vi "UI(Simple).vi"() -> (0 "error out":errorcluster)   [LabVIEW 2017, in "UI.lvlib"]
doc: "The Queued Message Handler of a Worker."
uses:
  UI.lvlib
  _support/UI State.ctl
  1af51285-6659-428e-9c15-de70f1a207c9.vi
  1756710f-d813-4077-a3f9-6f06171a4225.vi
  b1498353-a107-4479-98d0-7e76c0451ff6.vi
  242d01f8-d211-4c25-bb6c-8191a2acbe42.vi
  <userlib>/_NEVSTOP/Communicable State Machine(CSM)/_Polymophic/Add State(s) to Queue By BOOL(Element).vi
  <userlib>/_NEVSTOP/Communicable State Machine(CSM)/AdvanceAPI/CSM - Revert Arguments-Safe String.vi
  <userlib>/_NEVSTOP/Communicable State Machine(CSM)/AdvanceAPI/CSM - Make String Arguments Safe.vi
  <userlib>/_NEVSTOP/Communicable State Machine(CSM)/AdvanceAPI/CSM - Break Down Multiple States String.vi
  <userlib>/_NEVSTOP/Communicable State Machine(CSM)/AdvanceAPI/CSM - Keywords.vi
  <userlib>/_NEVSTOP/Communicable State Machine(CSM)/addons/INI-Static-Variable-Support/_Support/instances/_CSM - Read File Logger Configuration - v1.0.vi
  <userlib>/_NEVSTOP/Communicable State Machine(CSM)/_Shared/Trim Single-line Text.vi
  <userlib>/_NEVSTOP/Communicable State Machine(CSM)/addons/API-String-Arugments-Support/_Support/Convert API String Arguments to Data(variant).vi
  <userlib>/_NEVSTOP/Communicable State Machine(CSM)/addons/API-String-Arugments-Support/_Support/Query Data as API String Arguments(variant).vi
  <userlib>/_NEVSTOP/Communicable State Machine(CSM)/addons/MassData-Parameter/_support/FGV-MassData.vi
  Acquisition/Acquisition.lvlib
  Logging/Logging.lvlib
  <userlib>/_NEVSTOP/Communicable State Machine(CSM)/Communicable State Machine.lvlib
  <userlib>/_NEVSTOP/Communicable State Machine(CSM)/addons/MassData-Parameter/CSM MassData Parameter Support.lvlib
  <userlib>/_NEVSTOP/Communicable State Machine(CSM)/addons/INI-Static-Variable-Support/INI-Static-Variable-Support.lvlib
  <userlib>/_NEVSTOP/Communicable State Machine(CSM)/addons/Logger/CSM File Logger.lvlib
  <userlib>/_NEVSTOP/Communicable State Machine(CSM)/addons/Watchdog/CSM Watchdog.lvlib
  <userlib>/_NEVSTOP/Communicable State Machine(CSM)/_Polymophic/Build Synchronous Message with Arguments.vi
panel:
  out "WaveformGraph":waveform(dbl)[](graph)
  in  "Settings":bool
  in  "Start":bool
  in  "Stop":bool
  out "Status":string
  in  "Exit":bool
  # "Continuous Measurement and Data Logger - CSM Version"
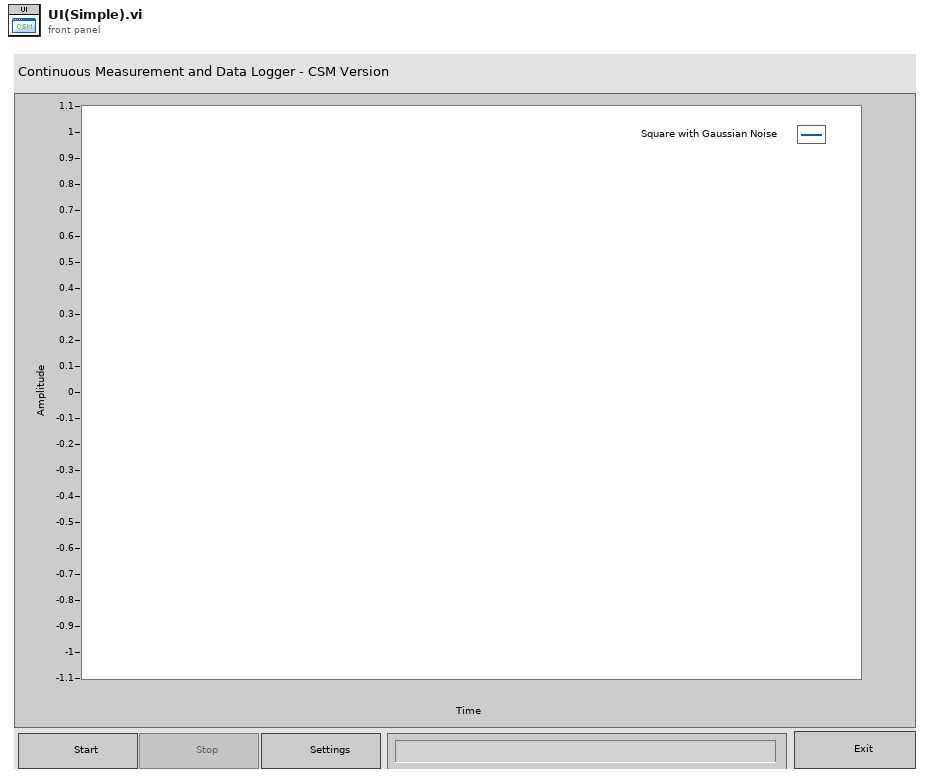
[diagram p1: front panel]
types:
  T1 = cluster{"Enable":bool, "Limit":cluster{"FileSize":i64, "FileNum":i32}, "Timestamp.Format":string, "AutoExit":bool}
  T2 = enum32{"Invalid", "Standard", "Closed", "Hidden", "Minimized", "Maximized"}
  T3 = enum32{"invalid app kind", "Development System", "Run Time System", "Student Edition", "Embedded LabVIEW", "Evaluation", "Custom"}
  T4 = typedef "UI.lvlib/UI State.ctl" = enum16{"Idle", "Acquiring and Logging", "Waiting for Exit", "Waiting for Exit (Acq Stopped)", "Waiting for Exit (Log Stopped)", "Waiting for Stop", "Waiting for Stop (Acq Stopped)", "Waiting for Stop (Log Stopped)"}
  T5 = enum32{"Invalid", "Default", "Floating", "Floating/Auto-Hide", "Modal"}
  T6 = typedef "Communicable State Machine.lvlib/_CSM_Response Source Message.ctl" = cluster{"‘State":string, "’Arguments":string, "’Error":errorcluster}
  T7 = cluster{"Current VI Reference":refnum<vi>, "Close Panel on Exit?":bool}
  T8 = cluster{"Core":cluster{"Current VI Reference":refnum<vi>, "Close Panel on Exit?":bool}, "UI Refs":cluster{"Start Ref":refnum<vi>, "Stop Ref":refnum<vi>, "Settings Ref":refnum<vi>, "Exit Ref":refnum<vi>, "Status Ref":refnum<vi>, "Data Ref":refnum<vi>, "Data Source Ref":refnum<vi>}, "State":T4, "Relationships":string}
  T9 = cluster{"Start Ref":refnum<vi>, "Stop Ref":refnum<vi>, "Settings Ref":refnum<vi>, "Exit Ref":refnum<vi>, "Status Ref":refnum<vi>, "Data Ref":refnum<vi>, "Data Source Ref":refnum<vi>}
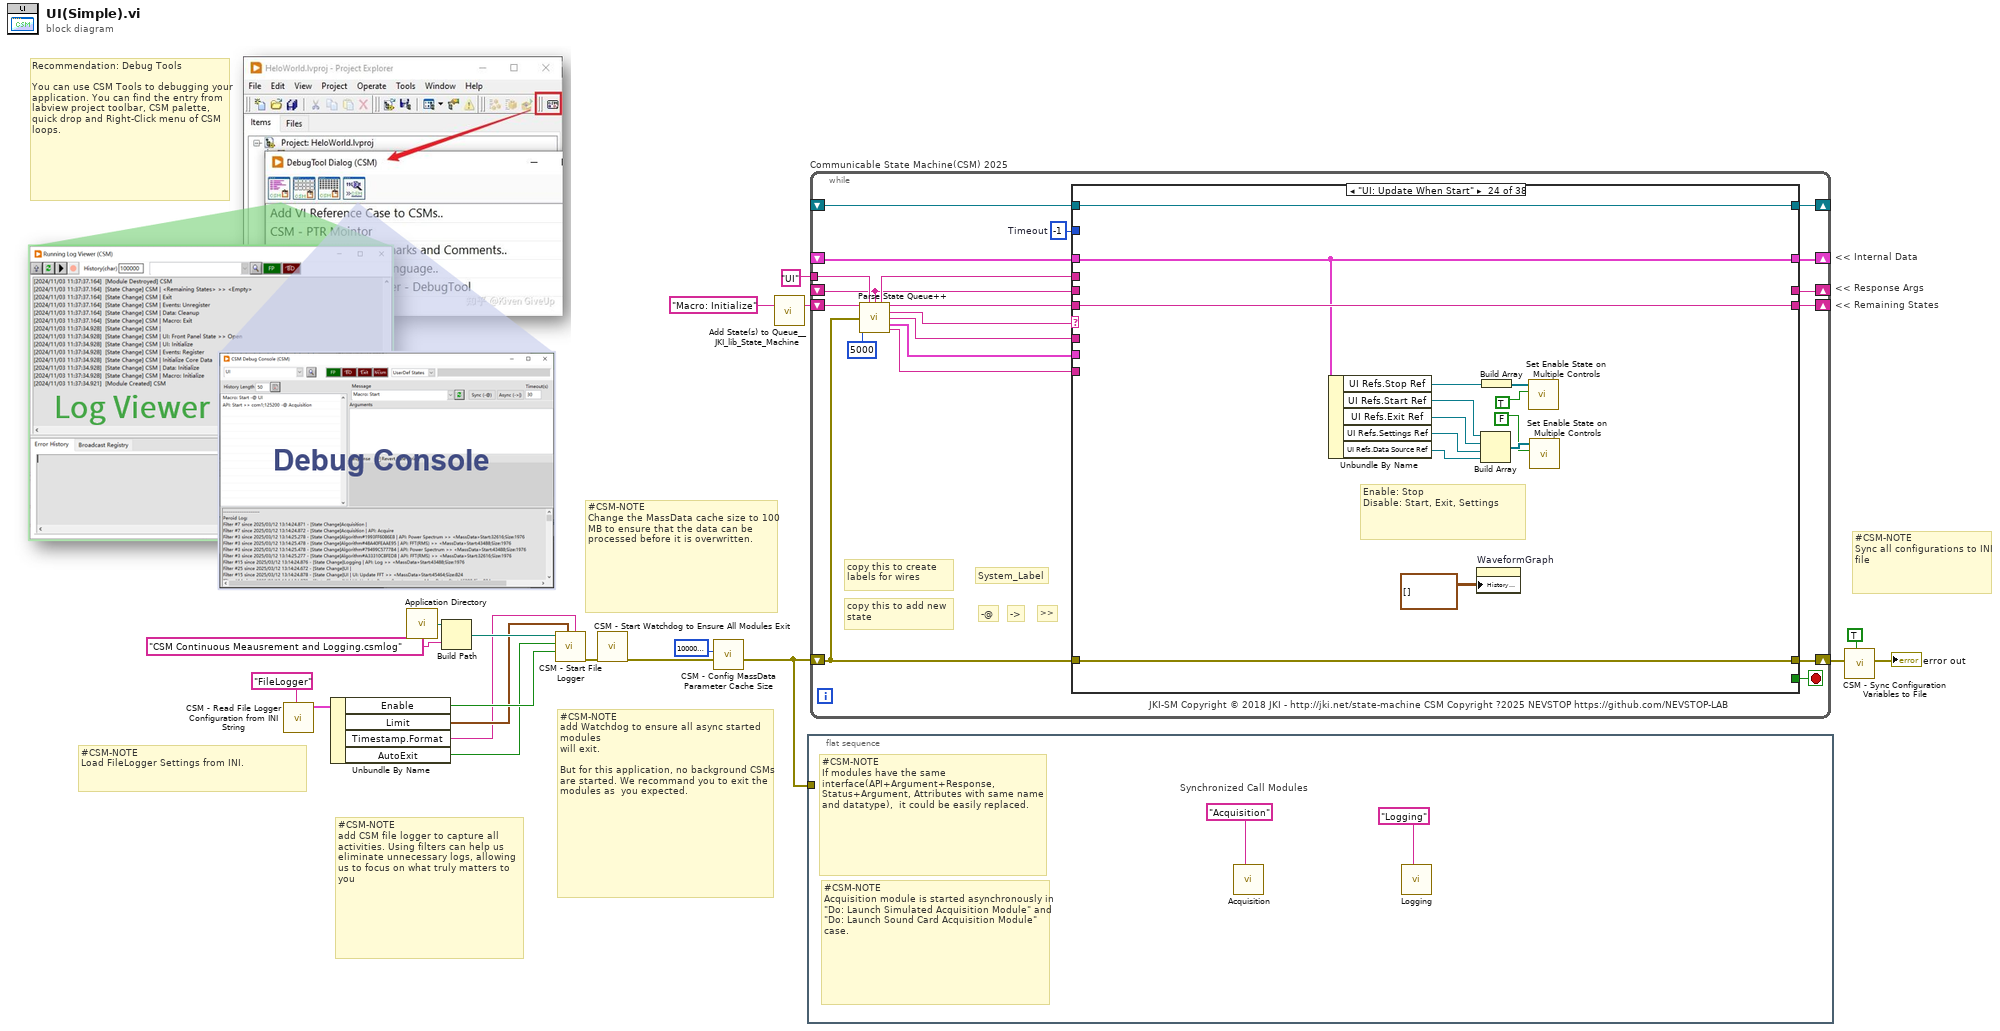
[diagram p0: block diagram]
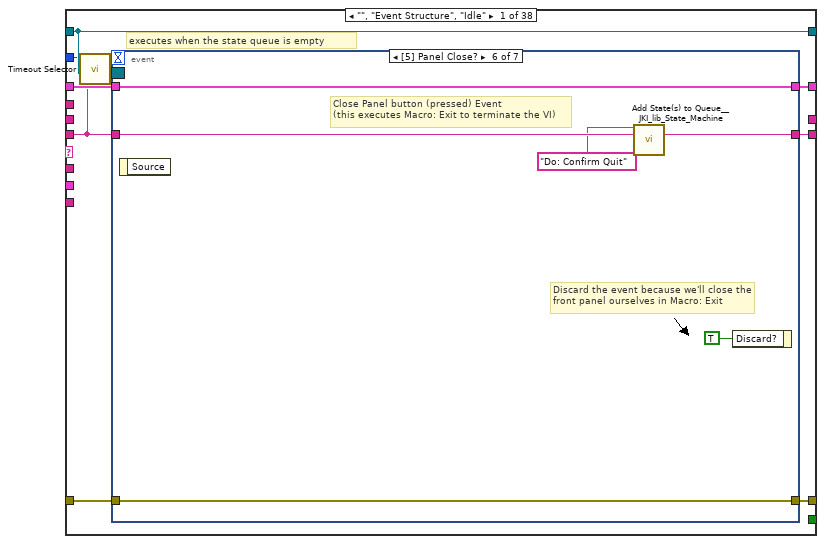
[diagram p2: hidden frame]
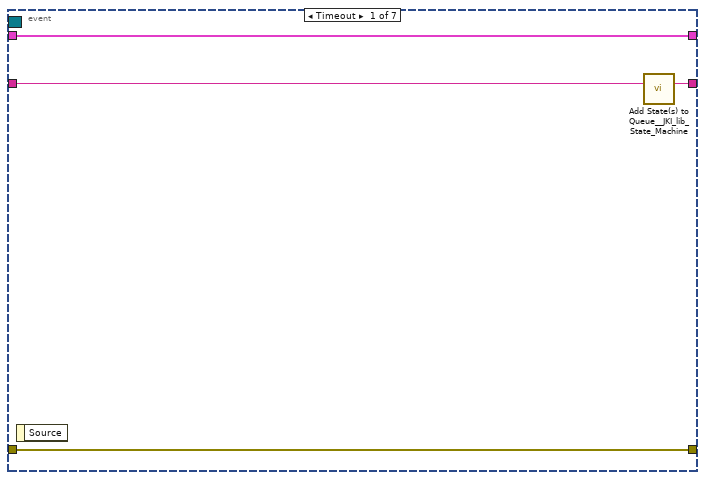
[diagram p3: hidden frame]
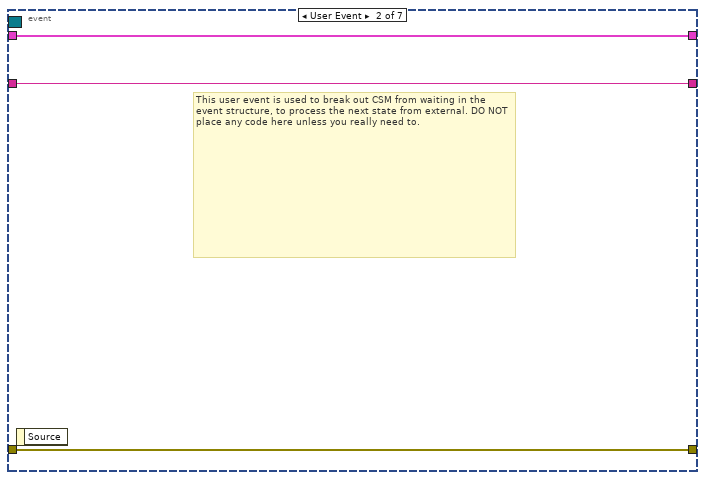
[diagram p4: hidden frame]
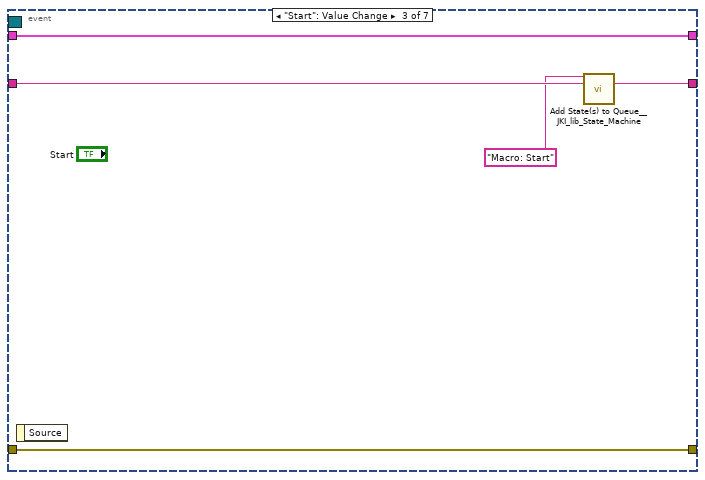
[diagram p5: hidden frame]
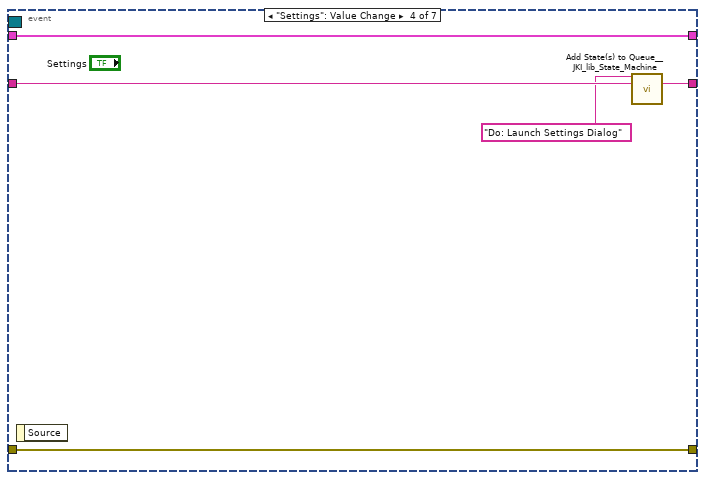
[diagram p6: hidden frame]
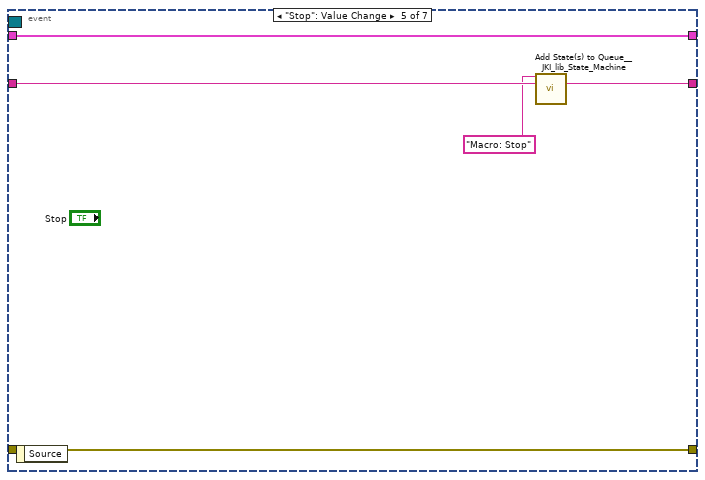
[diagram p7: hidden frame]
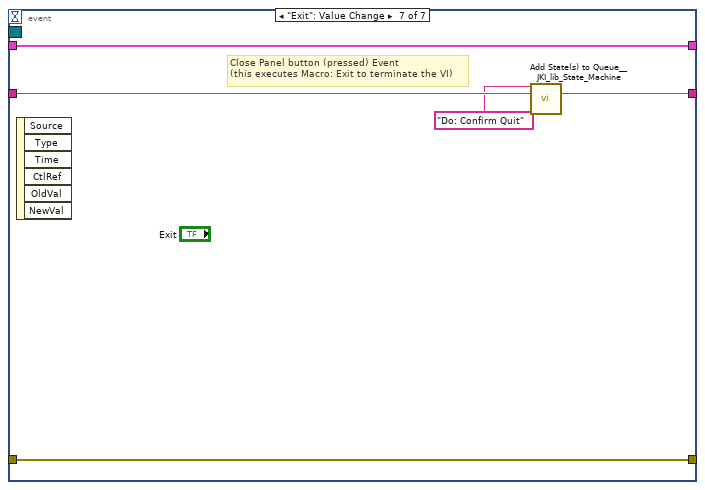
[diagram p8: hidden frame]
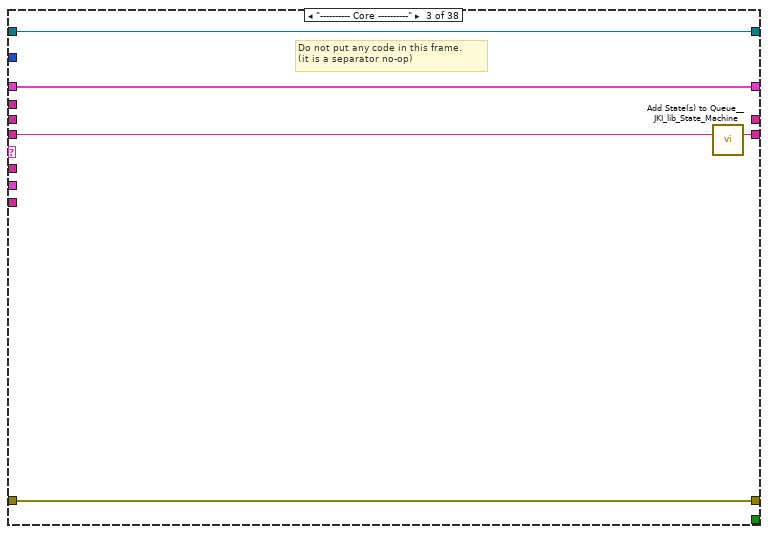
[diagram p10: hidden frame]
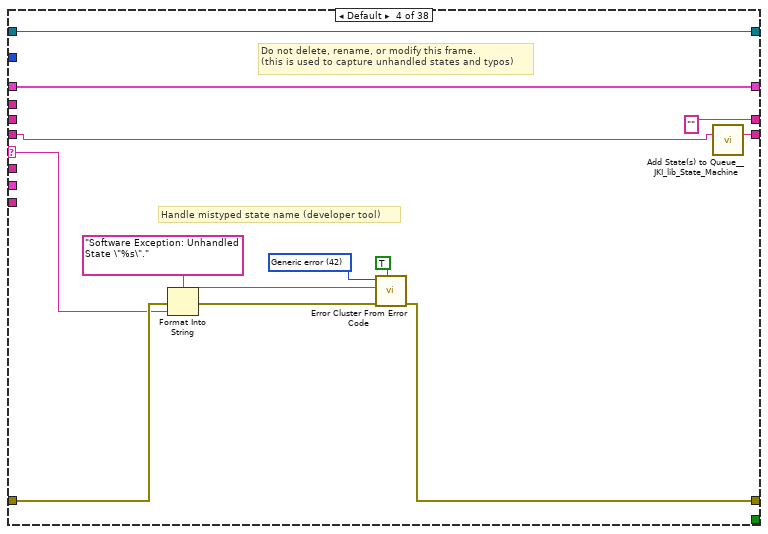
[diagram p11: hidden frame]
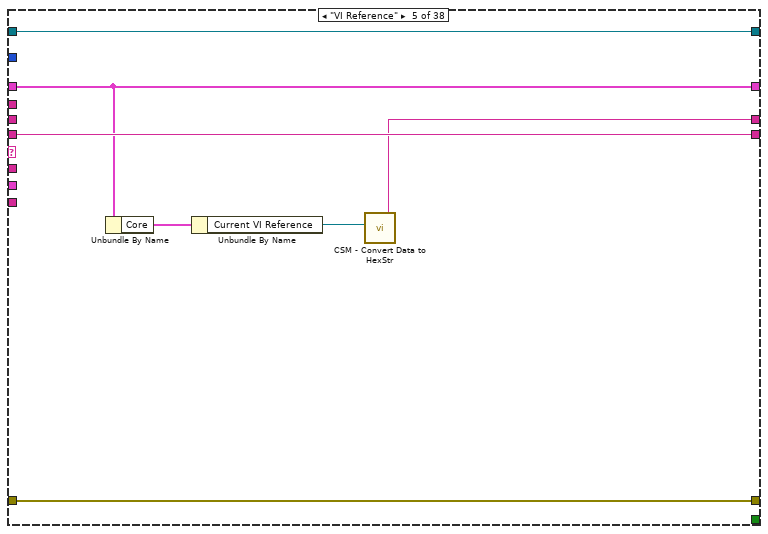
[diagram p12: hidden frame]
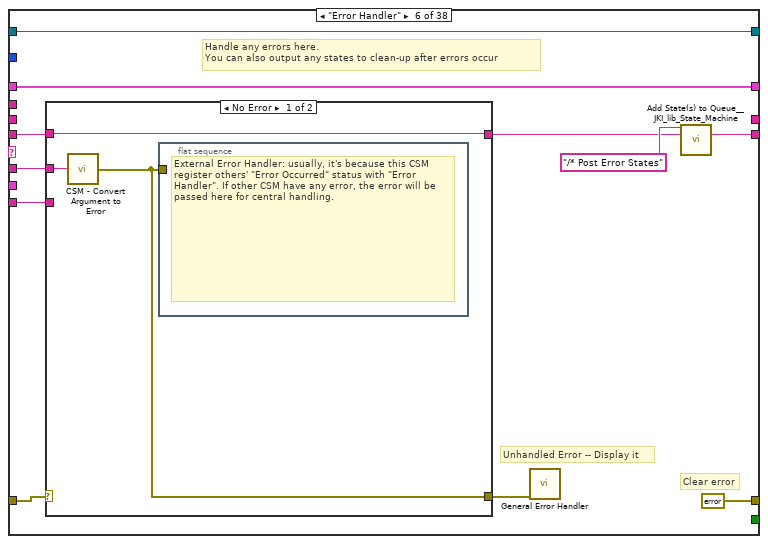
[diagram p13: hidden frame]
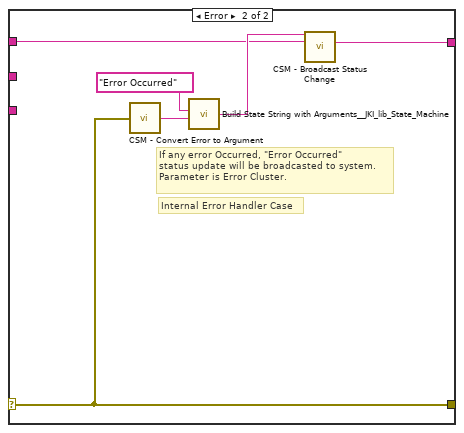
[diagram p14: hidden frame]
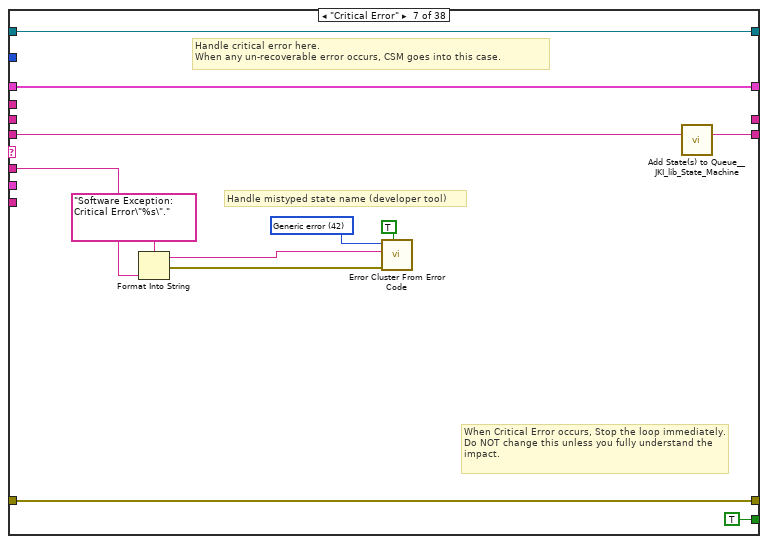
[diagram p15: hidden frame]
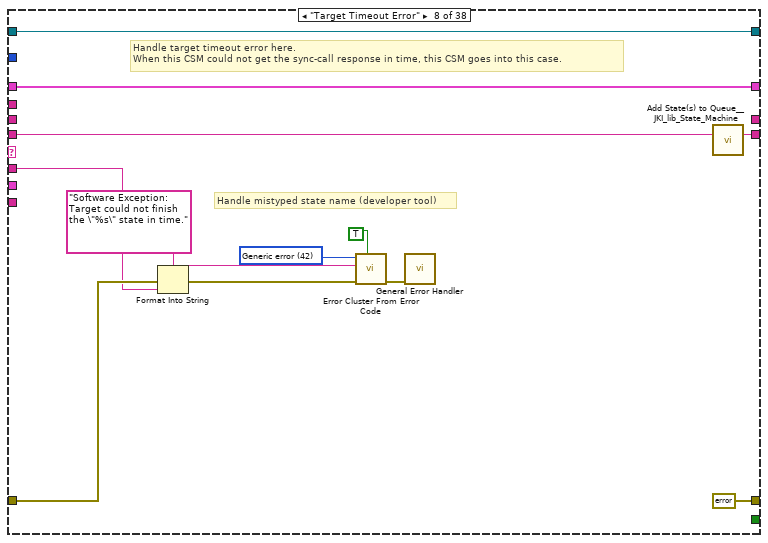
[diagram p16: hidden frame]
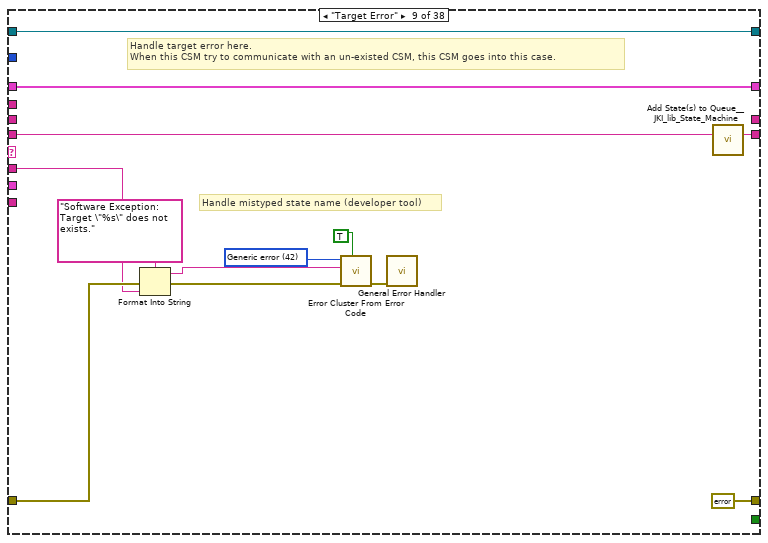
[diagram p17: hidden frame]
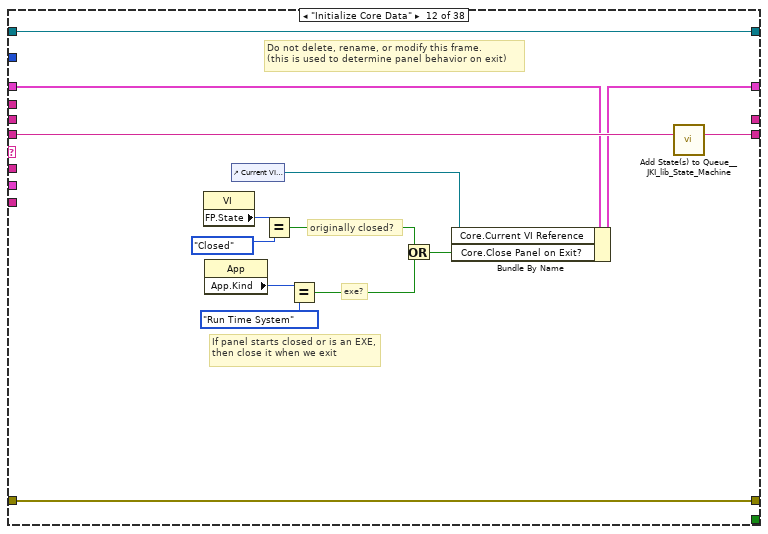
[diagram p20: hidden frame]
diagram:
  # "#CSM-NOTE\nSync all configurations to INI file"
  # "#CSM-NOTE\nChange the MassData cache size to 100 MB to ensure that the data can be processed before it is overwritten."
  # "Recommendation: Debug Tools\n\nYou can use CSM Tools to debugging your application. You can find the entry from labview project toolbar, CSM palette, quick drop and Right-Click menu of CSM loops."
  # "#CSM-NOTE\nLoad FileLogger Settings from INI."
  # "#CSM-NOTE\nadd CSM file logger to capture all activities. Using filters can help us eliminate unnecessary logs, allowing us to focus on what truly matters to you"
  # "#CSM-NOTE\nadd Watchdog to ensure all async started modules\nwill exit. \n\nBut for this application, no background CSMs are started. We recommand you to exit the modules as  you expected."
  # "<< Internal Data"
  # "<< Response Args"
  # "<< Remaining States"
  n1 = call-poly <userlib>:"CSM - Read File Logger Configuration from INI String.vi"("Section Name(\"FileLogger\")"="FileLogger" ("Section Name(\"\" as Default)")) -> ("FileLogger Configuration-v1"=w11:T1)  [unwired: 7 in, 1 out]
  n2 = Unbundle By Name(w11) -> ("Enable"=w10:bool, "Limit"=w9:cluster{"FileSize":i64, "FileNum":i32}, "Timestamp.Format"=w7:string, "AutoExit"=w8:bool)
  n3 = call <vilib>:"Application Directory.vi"() -> ("Application Directory"=w16:path)
  n4 = Build Path(base path=w16, name or relative path="CSM Continuous Meausrement and Logging.csmlog") -> (appended path=w14:path)
  n5 = call <userlib>:"CSM - Start File Logger.vi"("Timestamp format"=w7, "log limit"=w9, "WatchDog? (T)"=w10, "Exit When All Module Exist?(F)"=w8, "Log File Path"=w14) -> ("Error out"=w13:errorcluster)  [unwired: 4 in, 2 out]
  n6 = call <userlib>:"CSM - Start Watchdog to Ensure All Modules Exit.vi"("error in (no error)"=w13) -> ("error out"=w5:errorcluster)  [unwired: 10 in]
  n7 = call <userlib>:"CSM - Config MassData Parameter Cache Size.vi"("Error in"=w5, "size(1M)"=100000000) -> ("Error out"=w4:errorcluster)  [unwired: 9 in]
  n8 = call <vilib>:"Add State(s) to Queue__JKI_lib_State_Machine.vi"("State(s) in (\"\")"="Macro: Initialize") -> ("States Out"=w17:string)  [unwired: 14 in]
  n9 = flat-sequence {
    tunnel: w4 -> [_]
    frame #0 {
      # "Synchronized Call Modules"
      # "#CSM-NOTE\nAcquisition module is started asynchronously in \"Do: Launch Simulated Acquisition Module\" and \"Do: Launch Sound Card Acquisition Module\" case."
      # "#CSM-NOTE\nIf modules have the same interface(API+Argument+Response, Status+Argument, Attributes with same name and datatype),  it could be easily replaced."
      n10 = call "Acquisition.vi"("Name(\"\" to use uuid)"="Acquisition" ("Name(\"\" to use uuid)")) -> ()  [unwired: 11 in]
      n11 = call "Logging.vi"("Name(\"\" to use uuid)"="Logging" ("Name(\"\" to use uuid)")) -> ()  [unwired: 11 in]
    }
  }
  n12 = while "Communicable State Machine(CSM) 2025" {
    shift-right: [w36] -> _
    shift-left: _ -> [w35]
    shift-right: [w39] -> w2
    shift-left: w4 -> [w33]
    shift-right: [w38] -> _
    shift-left: w17 -> [w40]
    tunnel: "UI" ("Name(\"\" to use uuid)") -> [w28]
    shift-right: [w31] -> _
    shift-left: _ -> [w23]
    shift-right: [w30] -> _
    shift-left: _ -> [w29]
    stop <- w37 stop-if-true
    w34 = -1  # Timeout
    # "JKI-SM Copyright © 2018 JKI - http://jki.net/state-machine CSM Copyright ?2025 NEVSTOP https://github.com/NEVSTOP-LAB"
    # "copy this to add new state"
    # ">>"
    # "->"
    # "-@"
    # "copy this to create labels for wires"
    # "System_Label"
    n13 = call <userlib>:"Parse State Queue++.vi"("State Queue"=w40, "Name(\"\" to use uuid)"=w28, "Response Arguments"=w23, "Previous Error"=w33, "Response Timeout(-2 use global Settings)"=5000 ("Response Timeout(1000ms)")) -> ("Name Used"=w24:string, "Remaining States"=w41:string, "Current State"=w27:string, "Arguments"=w22:string, ">> Response Source Message >>"=w26:T6, ">> Source CSM >>"=w25:string)  [unwired: 5 in]
    n14 = case shown="\"UI: Update When Start\"" w27 {
      selector: w27 -> [_ _ _ w95 _ _ _ _ _ _ _ _ _ _ _ _ _ _ _ _ _ _ _ _ _ _ _ _ _ _ _ _ _ _ _ _ _ _]
      tunnel: w41 -> [w42 w86 w92 w99 w111 w116 w142 w152 w165 w173 w177 w192 w199 w204 w213 w219 w226 w233 w238 w244 w248 w254 w271 w284 w297 w305 w321 w395 w404 w415 w422 w424 w435 w452 w471 w477 w485 w523]
      tunnel: w22 -> [_ _ _ _ _ w114 w135 w148 w161 _ _ _ _ _ _ w217 w223 _ _ _ _ _ _ _ _ w300 w315 w390 w408 _ _ _ _ _ _ w472 _ _]
      tunnel: w35 -> [w49 w85 w89 w97 w110 w122 w143 w150 w163 w172 w176 w185 w197 w201 _ w216 w224 w228 w235 w243 w247 w251 w258 w274 w287 w303 w317 w393 w410 w412 w419 w427 w431 w450 w468 w474 w478 w518]
      tunnel: [w48 w87 w90 w101 w112 errorcluster {"status"=FALSE, "code"=0, "source"=""} ("error out") w144 errorcluster {"status"=FALSE, "code"=0, "source"=""} ("error out") errorcluster {"status"=FALSE, "code"=0, "source"=""} ("error out") w174 w178 w189 w196 w202 w207 w215 w222 w229 w236 w239 w246 w252 w269 w285 w298 w301 w318 w387 w406 w413 w420 w430 w439 _ w469 w475 w479 _] -> w39
      tunnel: w33 -> [w47 w87 w90 w100 w112 w120 w144 w153 w166 w174 w178 w189 w196 w202 w207 _ _ w230 w236 _ w249 w252 w269 w285 w298 w302 w319 _ _ w413 w420 w430 w439 _ w469 w475 _ _]
      tunnel: [w50 w86 w91 w98 w111 w118 w141 w151 w164 w173 w177 w191 w198 w203 w212 w219 w226 w232 w237 w244 w248 w253 w270 w284 w297 w304 w320 w395 w405 w414 w421 w425 w436 w451 w470 w476 w485 w516] -> w38
      tunnel: [_ _ _ _ _ _ TRUE _ _ _ _ _ TRUE _ _ _ _ _ _ _ _ _ _ _ _ _ _ _ _ _ _ _ _ _ _ _ _ _] -> w37
      tunnel: [w46 w85 w89 w97 w110 w122 w143 w150 w163 w172 w176 w190 w197 w201 w206 w214 w220 w228 w235 w243 w247 w251 w257 w274 w287 w303 w317 w393 w410 w412 w419 w426 w437 w450 w468 w474 w478 w517] -> w36
      tunnel: w34 -> [w44 _ _ _ _ _ _ _ _ _ _ _ _ _ _ _ _ _ _ _ _ _ _ _ _ _ _ _ _ _ _ _ _ _ _ _ _ _]
      tunnel: w25 -> [_ _ _ _ _ w113 _ _ _ _ _ _ _ _ _ _ _ _ _ _ _ _ _ _ _ _ _ _ _ _ _ _ _ _ _ _ _ _]
      tunnel: w26 -> [_ _ _ _ _ _ _ _ _ _ _ _ _ _ _ _ _ _ _ _ _ _ _ _ _ _ _ _ _ _ _ _ _ _ _ _ _ _]
      tunnel: [_ _ _ "" w106 _ _ _ _ _ _ _ _ _ _ _ w221 _ _ _ _ _ _ _ _ _ _ _ _ _ _ _ _ _ _ _ _ _] -> w31
      tunnel: [w45 w84 w88 w93 w109 w121 w133 w147 w160 w171 w175 w179 w194 w200 w210 w218 w225 w227 w234 w242 w245 w250 w268 w283 w296 w299 w314 w394 w409 w411 w418 w429 w438 w443 w467 w473 w486 w522] -> w30
      tunnel: w29 -> [w45 w84 w88 w93 w109 w121 w133 w147 w160 w171 w175 w179 w194 w200 w210 w218 w225 w227 w234 _ w245 w250 w268 w283 w296 w299 w314 w394 w409 w411 w418 w429 w438 w443 w467 w473 w486 w522]
      tunnel: w24 -> [_ _ _ _ _ _ _ _ _ _ _ _ _ _ _ _ _ _ _ w241 _ _ _ _ _ _ _ _ _ _ _ _ _ _ _ _ w481 _]
      tunnel: w23 -> [_ _ _ _ _ _ _ _ _ _ _ _ _ _ _ _ _ _ _ _ _ _ _ _ _ _ _ _ _ _ _ _ _ _ _ _ _ _]
      frame "", "Event Structure", "Idle" {
        # "executes when the state queue is empty"
        n15 = call <userlib>:"Timeout Selector.vi"("Remaining States"=w42, "Timeout Expected"=w44) -> ("Timeout"=w43:i32)  [unwired: 5 in]
        n16 = event shown="[5] Panel Close?" {
          selector: w45 -> [_ _ _ _ _ _ _]
          dyn-events: _ -> [_ _ _ _ _ _ _]
          timeout: w43 -> [_ _ _ _ _ _ _]
          tunnel: w42 -> [w54 w56 w59 w64 w69 w78 w83]
          tunnel: [w53 w56 w60 w65 w70 w77 w82] -> w50
          tunnel: w49 -> [w51 w57 w61 w66 w71 w75 w80]
          tunnel: [w52 w55 w62 w67 w72 w76 w81] -> w48
          tunnel: w47 -> [w52 w55 w62 w67 w72 w76 w81]
          tunnel: [w51 w57 w61 w66 w71 w75 w80] -> w46
          event Timeout {
            n17 = event-data() -> ()  [unwired: 1 in, 1 out]
            n18 = call <vilib>:"Add State(s) to Queue__JKI_lib_State_Machine.vi"("State(s) in (\"\")"=w54) -> ("States Out"=w53:string)  [unwired: 14 in]
          }
          event User Event {
            # "This user event is used to break out CSM from waiting in the event structure, to process the next state from external. DO NOT place any code here unless you really need to."
            n19 = event-data() -> ()  [unwired: 1 in, 1 out]
          }
          event "Start": Value Change {
            n20 = event-data() -> ()  [unwired: 1 in, 1 out]
            n21 = call <vilib>:"Add State(s) to Queue__JKI_lib_State_Machine.vi"("State(s) in Front (\"\")"="Macro: Start" ("State(s) in Front (\"\")"), "State(s) in (\"\")"=w59) -> ("States Out"=w60:string)  [unwired: 13 in]
          }
          event "Settings": Value Change {
            n22 = event-data() -> ()  [unwired: 1 in, 1 out]
            n23 = call <vilib>:"Add State(s) to Queue__JKI_lib_State_Machine.vi"("State(s) in Front (\"\")"="Do: Launch Settings Dialog" ("State(s) in Front (\"\")"), "State(s) in (\"\")"=w64) -> ("States Out"=w65:string)  [unwired: 13 in]
          }
          event "Stop": Value Change {
            n24 = event-data() -> ()  [unwired: 1 in, 1 out]
            n25 = call <vilib>:"Add State(s) to Queue__JKI_lib_State_Machine.vi"("State(s) in Front (\"\")"="Macro: Stop" ("State(s) in Front (\"\")"), "State(s) in (\"\")"=w69) -> ("States Out"=w70:string)  [unwired: 13 in]
          }
          event Panel Close? {
            # "Discard the event because we'll close the front panel ourselves in Macro: Exit"
            # "Close Panel button (pressed) Event\n(this executes Macro: Exit to terminate the VI)"
            n26 = event-data() -> ()  [unwired: 1 in, 1 out]
            n27 = call <vilib>:"Add State(s) to Queue__JKI_lib_State_Machine.vi"("State(s) in Front (\"\")"="Do: Confirm Quit", "State(s) in (\"\")"=w78) -> ("States Out"=w77:string)  [unwired: 13 in]
            n28 = event-data("Discard?"=TRUE) -> ()  [unwired: 1 in, 1 out]
          }
          event "Exit": Value Change {
            # "Close Panel button (pressed) Event\n(this executes Macro: Exit to terminate the VI)"
            n29 = event-data() -> ()  [unwired: 1 in, 6 out]
            n30 = call <vilib>:"Add State(s) to Queue__JKI_lib_State_Machine.vi"("State(s) in Front (\"\")"="Do: Confirm Quit", "State(s) in (\"\")"=w83) -> ("States Out"=w82:string)  [unwired: 13 in]
          }
        }
      }
      frame "CSM Documentation" {
        # "CSM Documentation"
        # "State Syntax:\nStateCategory: State >> Argument -@ CSMName\nStateCategory: State >> Argument -> CSMName\n\nLine Terminator: Line feed"
        # "Commenting:\nTo add a comment use \"//\" or \"#\" and all text to the right will be ignored\nCommenting Example:\nUI: Initialize // This initializes the UI\n// Another comment line"
        # "Example:\nUI: Help >> About -@Main\nUI: Help >> About ->Main\n\nWhere \"UI\" is the state category\nWhere \"Help\" is the state\nWhere \"About\" is the argument\nWhere \"Main\" is the Name of CSM,which actually run the \"UI: Help >> About\"\n\n    \"-@\" stands for sync state. Current CSM will wait until the state is finished. \n            - if \"Main\" named CSM does not exist, \"Target Error\" will occur.\n            - if \"Main\" named CSM is in another sync remote state, \"Target Busy Error\" will occur.\n            - if \"Main\" named CSM could not finish the state in time, \"Target Timeout Error\" will occur.\n            - if everything is right. \"Response\" will occur with Argument back from \"Main\" named CSM. \n\n    \"->\" stands for async state. Current CSM will post the state and continue to next state in next iteration.\n            - if \"Main\" named CSM does not exist, \"Target Error\" will occur.\n            - if everything is right. \"Async Message Posted\" will occur.\n            - After State is finished. Caller will receive a \"Async Response\" state from callee.\n\nWhen duplicated name is used for multiple CSM module or some framework problem happens, \"Critical Error\" will occur."
      }
      frame "---------- Core ----------" {
        # "Do not put any code in this frame.\n(it is a separator no-op)"
        n31 = call <vilib>:"Add State(s) to Queue__JKI_lib_State_Machine.vi"("State(s) in (\"\")"=w92) -> ("States Out"=w91:string)  [unwired: 14 in]
      }
      frame Default {
        w104 = 42 items=["No error", "Argument error", "Memory is full", "Out of zone", "End of file", "File already open", "Generic file I/O error", "File not found", "File permission error", "Disk is full", "Duplicate path", "Too many files open", "System feature not enabled", "Resource file not found", "Cannot add resource", "Resource not found", "Image not found", "Image memory error", "Pen does not exist", "Config type invalid", "Config token not found", "Config parse error", "Config memory error", "Bad external code format", "Bad external code offset", "External code not present", "Null window", "Destroy window error", "Null menu", "Print aborted", "Bad print record", "Print driver error", "Windows error during printing", "Memory error during printing", "Print dialog error", "Generic print error", "Invalid device refnum", "Device not found", "Device parameter error", "Device unit error", "Cannot open device", "Device call aborted", "Generic error", "Cancelled by user", "Object ID too low", "Object ID too high", "Object not in heap", "Unknown heap", "Unknown object (invalid DefProc)", "Unknown object (DefProc not in table)", "Message out of range", "Invalid (null) method", "Unknown message", "Manager call not supported", "Bad address", "Network operation in progress", "Network operation timed out", "Connection is busy", "Network attribute not supported", "Network error", "Address in use", "System out of memory", "Connection aborted", "Connection refused", "Not connected", "Already connected", "Connection closed", "Initialization error (interapplication manager)", "Bad occurrence", "Wait on unbound occurrence handler", "Occurrence queue overflow", "Datalog type conflict", "Unused", "Unrecognized type (interapplication manager)", "Memory corrupt", "Failed to make temporary DLL", "Old CIN version", "Drag socket not found", "Failed to load drop-object", "Failed to register OLE object", "Failed to release OLE object", "Format specifier type mismatch", "Unknown format specifier", "Too few format specifiers", "Too many format specifiers", "Scan failed", "Newer CIN version", "Error converting to variant", "Runtime menu error", "Password tampered", "Variant attribute not found", "Incompatible variant data type", "Event data is not available", "Event Store is not present", "Occurrence is not found", "Event Queue is not created", "Event info is not available", "Refnum passed is NULL", "Error retrieving Class GUID", "Error retrieving CoClass GUID", "Error retrieving TypeLib GUID.", "Bad built application magic bytes.", "Specific driver is different from the specific driver associated with the Logical Name.", "There is no session opened to the class driver.", "Max Error", "MAX - Error with config objects", "MAX - Error loading configuration", "MAX - Group not supported"]
        # "Do not delete, rename, or modify this frame.\n(this is used to capture unhandled states and typos)"
        # "Handle mistyped state name (developer tool)"
        n32 = Format Into String(format string="Software Exception: Unhandled State \"%s\"." ("message"), error in=w100, w95) -> (resulting string=w103:string, error out=w102:errorcluster)  [unwired: 1 in]
        n33 = call <vilib>:"Error Cluster From Error Code.vi"("show call chain? (False)"=TRUE, "error in (no error)"=w102, "error message (\"\")"=w103, "error code (0)"=w104) -> ("error out"=w101:errorcluster)  [unwired: 5 in]
        n34 = call <vilib>:"Add State(s) to Queue__JKI_lib_State_Machine.vi"("State(s) in (\"\")"=w99) -> ("States Out"=w98:string)  [unwired: 14 in]
      }
      frame "VI Reference" {
        n35 = Unbundle By Name(w110) -> ("Core"=w108:T7)
        n36 = Unbundle By Name(w108) -> ("Current VI Reference"=w107:refnum<vi>)
        n37 = call <userlib>:"CSM - Convert Data to HexStr.vi"("Variant"=w107) -> ("HEX String (0-9,A-F)"=w106:string)  [unwired: 8 in]
      }
      frame "Error Handler" {
        # "Unhandled Error -- Display it"
        # "Handle any errors here.\nYou can also output any states to clean-up after errors occur"
        # "Clear error"
        n38 = case shown="No Error" w120 {
          selector: w120 -> [_ w127]
          tunnel: [w125 w129] -> w117
          tunnel: w116 -> [w125 w128]
          tunnel: [w124 w127] -> w115
          tunnel: w114 -> [w126 _]
          tunnel: w113 -> [_ _]
          frame No Error {
            n39 = call <userlib>:"CSM - Convert Argument to Error.vi"("Argument"=w126) -> ("error"=w124:errorcluster)  [unwired: 4 in]
            n40 = flat-sequence {
              tunnel: w124 -> [_]
              frame #0 {
                # "External Error Handler: usually, it's because this CSM register others' \"Error Occurred\" status with \"Error Handler\". If other CSM have any error, the error will be passed here for central handling."
              }
            }
          }
          frame Error {
            # "Internal Error Handler Case"
            # "If any error Occurred, \"Error Occurred\" \nstatus update will be broadcasted to system.\nParameter is Error Cluster."
            n41 = call <userlib>:"CSM - Convert Error to Argument.vi"("error"=w127) -> ("Argument"=w131:string)  [unwired: 4 in]
            n42 = call <vilib>:"Build State String with Arguments__JKI_lib_State_Machine.vi"("Arguments (\"\")"=w131, "State"="Error Occurred" ("Status with Arguments")) -> ("State with Arguments"=w130:string)  [unwired: 4 in]
            n43 = call <userlib>:"CSM - Broadcast Status Change.vi"("Status with Arguments"=w130, "State Queue"=w128) -> ("Remaining States"=w129:string)  [unwired: 13 in]
          }
        }
        n44 = call <vilib>:"General Error Handler.vi"("error in (no error)"=w115) -> ()  [unwired: 10 in, 5 out]
        n45 = call <vilib>:"Add State(s) to Queue__JKI_lib_State_Machine.vi"("State(s) in Front (\"\")"="/* Post Error States", "State(s) in (\"\")"=w117) -> ("States Out"=w118:string)  [unwired: 13 in]
      }
      frame "Critical Error" {
        w139 = 42 items=["No error", "Argument error", "Memory is full", "Out of zone", "End of file", "File already open", "Generic file I/O error", "File not found", "File permission error", "Disk is full", "Duplicate path", "Too many files open", "System feature not enabled", "Resource file not found", "Cannot add resource", "Resource not found", "Image not found", "Image memory error", "Pen does not exist", "Config type invalid", "Config token not found", "Config parse error", "Config memory error", "Bad external code format", "Bad external code offset", "External code not present", "Null window", "Destroy window error", "Null menu", "Print aborted", "Bad print record", "Print driver error", "Windows error during printing", "Memory error during printing", "Print dialog error", "Generic print error", "Invalid device refnum", "Device not found", "Device parameter error", "Device unit error", "Cannot open device", "Device call aborted", "Generic error", "Cancelled by user", "Object ID too low", "Object ID too high", "Object not in heap", "Unknown heap", "Unknown object (invalid DefProc)", "Unknown object (DefProc not in table)", "Message out of range", "Invalid (null) method", "Unknown message", "Manager call not supported", "Bad address", "Network operation in progress", "Network operation timed out", "Connection is busy", "Network attribute not supported", "Network error", "Address in use", "System out of memory", "Connection aborted", "Connection refused", "Not connected", "Already connected", "Connection closed", "Initialization error (interapplication manager)", "Bad occurrence", "Wait on unbound occurrence handler", "Occurrence queue overflow", "Datalog type conflict", "Unused", "Unrecognized type (interapplication manager)", "Memory corrupt", "Failed to make temporary DLL", "Old CIN version", "Drag socket not found", "Failed to load drop-object", "Failed to register OLE object", "Failed to release OLE object", "Format specifier type mismatch", "Unknown format specifier", "Too few format specifiers", "Too many format specifiers", "Scan failed", "Newer CIN version", "Error converting to variant", "Runtime menu error", "Password tampered", "Variant attribute not found", "Incompatible variant data type", "Event data is not available", "Event Store is not present", "Occurrence is not found", "Event Queue is not created", "Event info is not available", "Refnum passed is NULL", "Error retrieving Class GUID", "Error retrieving CoClass GUID", "Error retrieving TypeLib GUID.", "Bad built application magic bytes.", "Specific driver is different from the specific driver associated with the Logical Name.", "There is no session opened to the class driver.", "Max Error", "MAX - Error with config objects", "MAX - Error loading configuration", "MAX - Group not supported"]
        # "Handle critical error here.\nWhen any un-recoverable error occurs, CSM goes into this case."
        # "When Critical Error occurs, Stop the loop immediately. Do NOT change this unless you fully understand the impact."
        # "Handle mistyped state name (developer tool)"
        n46 = Format Into String(format string="Software Exception: Critical Error\"%s\"." ("message"), w135) -> (resulting string=w138:string, error out=w137:errorcluster)  [unwired: 2 in]
        n47 = call <vilib>:"Error Cluster From Error Code.vi"("show call chain? (False)"=TRUE, "error in (no error)"=w137, "error message (\"\")"=w138, "error code (0)"=w139) -> ()  [unwired: 5 in, 1 out]
        n48 = call <vilib>:"Add State(s) to Queue__JKI_lib_State_Machine.vi"("State(s) in (\"\")"=w142) -> ("States Out"=w141:string)  [unwired: 14 in]
      }
      frame "Target Timeout Error" {
        w156 = 42 items=["No error", "Argument error", "Memory is full", "Out of zone", "End of file", "File already open", "Generic file I/O error", "File not found", "File permission error", "Disk is full", "Duplicate path", "Too many files open", "System feature not enabled", "Resource file not found", "Cannot add resource", "Resource not found", "Image not found", "Image memory error", "Pen does not exist", "Config type invalid", "Config token not found", "Config parse error", "Config memory error", "Bad external code format", "Bad external code offset", "External code not present", "Null window", "Destroy window error", "Null menu", "Print aborted", "Bad print record", "Print driver error", "Windows error during printing", "Memory error during printing", "Print dialog error", "Generic print error", "Invalid device refnum", "Device not found", "Device parameter error", "Device unit error", "Cannot open device", "Device call aborted", "Generic error", "Cancelled by user", "Object ID too low", "Object ID too high", "Object not in heap", "Unknown heap", "Unknown object (invalid DefProc)", "Unknown object (DefProc not in table)", "Message out of range", "Invalid (null) method", "Unknown message", "Manager call not supported", "Bad address", "Network operation in progress", "Network operation timed out", "Connection is busy", "Network attribute not supported", "Network error", "Address in use", "System out of memory", "Connection aborted", "Connection refused", "Not connected", "Already connected", "Connection closed", "Initialization error (interapplication manager)", "Bad occurrence", "Wait on unbound occurrence handler", "Occurrence queue overflow", "Datalog type conflict", "Unused", "Unrecognized type (interapplication manager)", "Memory corrupt", "Failed to make temporary DLL", "Old CIN version", "Drag socket not found", "Failed to load drop-object", "Failed to register OLE object", "Failed to release OLE object", "Format specifier type mismatch", "Unknown format specifier", "Too few format specifiers", "Too many format specifiers", "Scan failed", "Newer CIN version", "Error converting to variant", "Runtime menu error", "Password tampered", "Variant attribute not found", "Incompatible variant data type", "Event data is not available", "Event Store is not present", "Occurrence is not found", "Event Queue is not created", "Event info is not available", "Refnum passed is NULL", "Error retrieving Class GUID", "Error retrieving CoClass GUID", "Error retrieving TypeLib GUID.", "Bad built application magic bytes.", "Specific driver is different from the specific driver associated with the Logical Name.", "There is no session opened to the class driver.", "Max Error", "MAX - Error with config objects", "MAX - Error loading configuration", "MAX - Group not supported"]
        # "Handle target timeout error here.\nWhen this CSM could not get the sync-call response in time, this CSM goes into this case."
        # "Handle mistyped state name (developer tool)"
        n49 = Format Into String(format string="Software Exception: Target could not finish the \"%s\" state in time." ("message"), error in=w153, w148) -> (resulting string=w155:string, error out=w154:errorcluster)  [unwired: 1 in]
        n50 = call <vilib>:"Error Cluster From Error Code.vi"("show call chain? (False)"=TRUE, "error in (no error)"=w154, "error message (\"\")"=w155, "error code (0)"=w156) -> ("error out"=w145:errorcluster)  [unwired: 5 in]
        n51 = call <vilib>:"General Error Handler.vi"("error in (no error)"=w145) -> ()  [unwired: 10 in, 5 out]
        n52 = call <vilib>:"Add State(s) to Queue__JKI_lib_State_Machine.vi"("State(s) in (\"\")"=w152) -> ("States Out"=w151:string)  [unwired: 14 in]
      }
      frame "Target Error" {
        w169 = 42 items=["No error", "Argument error", "Memory is full", "Out of zone", "End of file", "File already open", "Generic file I/O error", "File not found", "File permission error", "Disk is full", "Duplicate path", "Too many files open", "System feature not enabled", "Resource file not found", "Cannot add resource", "Resource not found", "Image not found", "Image memory error", "Pen does not exist", "Config type invalid", "Config token not found", "Config parse error", "Config memory error", "Bad external code format", "Bad external code offset", "External code not present", "Null window", "Destroy window error", "Null menu", "Print aborted", "Bad print record", "Print driver error", "Windows error during printing", "Memory error during printing", "Print dialog error", "Generic print error", "Invalid device refnum", "Device not found", "Device parameter error", "Device unit error", "Cannot open device", "Device call aborted", "Generic error", "Cancelled by user", "Object ID too low", "Object ID too high", "Object not in heap", "Unknown heap", "Unknown object (invalid DefProc)", "Unknown object (DefProc not in table)", "Message out of range", "Invalid (null) method", "Unknown message", "Manager call not supported", "Bad address", "Network operation in progress", "Network operation timed out", "Connection is busy", "Network attribute not supported", "Network error", "Address in use", "System out of memory", "Connection aborted", "Connection refused", "Not connected", "Already connected", "Connection closed", "Initialization error (interapplication manager)", "Bad occurrence", "Wait on unbound occurrence handler", "Occurrence queue overflow", "Datalog type conflict", "Unused", "Unrecognized type (interapplication manager)", "Memory corrupt", "Failed to make temporary DLL", "Old CIN version", "Drag socket not found", "Failed to load drop-object", "Failed to register OLE object", "Failed to release OLE object", "Format specifier type mismatch", "Unknown format specifier", "Too few format specifiers", "Too many format specifiers", "Scan failed", "Newer CIN version", "Error converting to variant", "Runtime menu error", "Password tampered", "Variant attribute not found", "Incompatible variant data type", "Event data is not available", "Event Store is not present", "Occurrence is not found", "Event Queue is not created", "Event info is not available", "Refnum passed is NULL", "Error retrieving Class GUID", "Error retrieving CoClass GUID", "Error retrieving TypeLib GUID.", "Bad built application magic bytes.", "Specific driver is different from the specific driver associated with the Logical Name.", "There is no session opened to the class driver.", "Max Error", "MAX - Error with config objects", "MAX - Error loading configuration", "MAX - Group not supported"]
        # "Handle target error here.\nWhen this CSM try to communicate with an un-existed CSM, this CSM goes into this case."
        # "Handle mistyped state name (developer tool)"
        n53 = Format Into String(format string="Software Exception: Target \"%s\" does not exists." ("message"), error in=w166, w161) -> (resulting string=w168:string, error out=w167:errorcluster)  [unwired: 1 in]
        n54 = call <vilib>:"Error Cluster From Error Code.vi"("show call chain? (False)"=TRUE, "error in (no error)"=w167, "error message (\"\")"=w168, "error code (0)"=w169) -> ("error out"=w159:errorcluster)  [unwired: 5 in]
        n55 = call <vilib>:"General Error Handler.vi"("error in (no error)"=w159) -> ()  [unwired: 10 in, 5 out]
        n56 = call <vilib>:"Add State(s) to Queue__JKI_lib_State_Machine.vi"("State(s) in (\"\")"=w165) -> ("States Out"=w164:string)  [unwired: 14 in]
      }
      frame "Async Response", "Response" {
        # "Handle Async-call Response (\"Async Response\" for ->)"
        # "Handle Sync-call Response (\"Response\" for -@)"
        # "After Message is executed, CSM+ goes to this state for receive the response. \n    For Async Message(->), \"Async Response\" is used. This CSM will goes to \"Async Message Posted\" immediately and receive the \"Async Response\" after the callee finishes the message.\n    For Sync Message(@),  This CSM will wait until the message is done and immediately goes to \"Response\""
      }
      frame "Async Message Posted" {
        # "Handle post action for async message (->)."
        # "After Async Message is posted (->), CSM+ goes to this state for post-action. You can use Argument - State to tell which Async Message is called."
      }
      frame "Initialize Core Data" {
        # "Do not delete, rename, or modify this frame.\n(this is used to determine panel behavior on exit)"
        # "originally closed?"
        # "exe?"
        # "If panel starts closed or is an EXE, then close it when we exit"
        n57 = property class="VI"() -> ("FP.State"=w182:T2)  [unwired: 2 in, 2 out]
        n58 = property class="App"() -> ("App.Kind"=w188:T3)  [unwired: 2 in, 2 out]
        n59 = control-ref of="Current VI Reference"() -> (w183:refnum<vi>)
        n60 = Equal?(x=w182, y=T2."Closed" ("Front Panel Window:State")) -> (x = y?=w180:bool)
        n61 = Equal?(x=w188, y=T3."Run Time System" ("Application:Kind")) -> (x = y?=w186:bool)
        n62 = Or(x=w180, y=w186) -> (x .or. y?=w184:bool)
        n63 = Bundle By Name(cluster=w185, "Core.Current VI Reference"=w183, "Core.Close Panel on Exit?"=w184) -> (w190:T8)
        n64 = call <vilib>:"Add State(s) to Queue__JKI_lib_State_Machine.vi"("State(s) in (\"\")"=w192) -> ("States Out"=w191:string)  [unwired: 14 in]
      }
      frame "Exit" {
        # "Do not put any code in this frame.\n(No errors that occur here will be handled.)"
        n65 = local write "Status"("Exit" ("Exit String")) -> ()
        n66 = call <vilib>:"Add State(s) to Queue__JKI_lib_State_Machine.vi"("State(s) in (\"\")"=w199) -> ("States Out"=w198:string)  [unwired: 14 in]
      }
      frame "---------- Data ----------" {
        # "Do not put any code in this frame.\n(It is a separator no-op. You can make a copy of this frame to create a new Data frame)"
        n67 = call <vilib>:"Add State(s) to Queue__JKI_lib_State_Machine.vi"("State(s) in (\"\")"=w204) -> ("States Out"=w203:string)  [unwired: 14 in]
      }
      frame "Data: Initialize" {
        w205 = ""  # Relationships
        w208 = UI_State."Idle"  # State
        w209 = T9 {"Start Ref"=refnum, "Stop Ref"=refnum, "Settings Ref"=refnum, "Exit Ref"=refnum, "Status Ref"=refnum, "Data Ref"=refnum, "Data Source Ref"=refnum}  # UI Refs
        w211 = T7 {"Current VI Reference"=refnum, "Close Panel on Exit?"=FALSE}  # Core
        # "Initialize the shift-register data, here.\n(data names are defined by what you wire into the bundle function)"
        n68 = Bundle("Core"=w211, "UI Refs"=w209, "State"=w208, "Relationships"=w205) -> (w206:T8)  [unwired: 1 in]
        n69 = call <vilib>:"Add State(s) to Queue__JKI_lib_State_Machine.vi"("State(s) in (\"\")"=w213) -> ("States Out"=w212:string)  [unwired: 14 in]
      }
      frame "Data: Set Configuration" {
        n70 = call "Convert API String Arguments to Data.vim"("Type"=w216, "String"=w217) -> ("error"=w215:errorcluster, "Data"=w214:T8)  [unwired: 6 in]
      }
      frame "Data: Get Configuration", "Data: Get Internal Data" {
        n71 = call "Query Data as API String Arguments.vim"("Setting Name"=w223, "Internal Data"=w224) -> ("error"=w222:errorcluster, "Setting as String"=w221:string, "Internal Data(dup)"=w220:T8)  [unwired: 7 in]
      }
      frame "Data: Cleanup" {
        # "Cleanup any data and references, here.\n(this is called automatically, by the Macro: Exit)"
        n72 = Unbundle By Name(w228) -> ("Core.Current VI Reference"=w231:refnum<vi>)
        n73 = Close Reference(reference=w231, error in (no error)=w230) -> (error out=w229:errorcluster)
        n74 = call <vilib>:"Add State(s) to Queue__JKI_lib_State_Machine.vi"("State(s) in (\"\")"=w233) -> ("States Out"=w232:string)  [unwired: 14 in]
      }
      frame "---------- Events ----------" {
        # "Do not put any code in this frame.\n(It is a separator no-op. You can make a copy of this frame to create a new UI frame)"
        n75 = call <vilib>:"Add State(s) to Queue__JKI_lib_State_Machine.vi"("State(s) in (\"\")"=w238) -> ("States Out"=w237:string)  [unwired: 14 in]
      }
      frame "Events: Register" {
        # "Register message event to break Waiting in Event structure."
        n76 = call <userlib>:"CSM - Get New State Notifier Event.vi"("Name(\"\" to use uuid) in"=w241) -> ("Error out"=w239:errorcluster, "New State Notifier Event"=w240:refnum<user-event>)  [unwired: 9 in]
        n77 = register-events(w240) -> (reference out=w242:refnum<event-registration>)  [unwired: 2 in, 1 out]
      }
      frame "Events: Unregister" {
        n78 = Unregister For Events(event registration refnum=w245, error in=w249) -> (error out=w246:errorcluster)
      }
      frame "---------- UI ----------" {
        # "Do not put any code in this frame.\n(It is a separator no-op. You can make a copy of this frame to create a new UI frame)"
        n79 = call <vilib>:"Add State(s) to Queue__JKI_lib_State_Machine.vi"("State(s) in (\"\")"=w254) -> ("States Out"=w253:string)  [unwired: 14 in]
      }
      frame "UI: Initialize" {
        # "Initialize the User Interface, here.\n(this is called automatically, by the Macro: Init)"
        n80 = control-ref of="WaveformGraph"() -> (w261:refnum<vi>)
        n81 = control-ref of="Start"() -> (w265:refnum<vi>)
        n82 = control-ref of="Stop"() -> (w255:refnum<vi>)
        n83 = control-ref of="Settings"() -> (w266:refnum<vi>)
        n84 = control-ref of="Exit"() -> (w267:refnum<vi>)
        n85 = control-ref of="Status"() -> (w262:refnum<vi>)
        n86 = Bundle By Name(cluster=w258, "UI Refs.Start Ref"=w265, "UI Refs.Stop Ref"=w255, "UI Refs.Settings Ref"=w266, "UI Refs.Exit Ref"=w267, "UI Refs.Status Ref"=w262, "UI Refs.Data Ref"=w261) -> (w257:T8)
        n87 = Build Array(w255) -> (w263:refnum<vi>[])
        n88 = Build Array(w265, w267, w266) -> (w264:refnum<vi>[])
        n89 = call "Set Enable State on Multiple Controls.vi"("Enable?"=TRUE, "Controls"=w264) -> ()  [unwired: 10 in]
        n90 = property on="WaveformGraph" class="WFChart (strict)"("History Data"=waveform(dbl)[][] []) -> ()  [unwired: 2 in, 2 out]
        n91 = call "Set Enable State on Multiple Controls.vi"("Enable?"=FALSE, "Controls"=w263) -> ()  [unwired: 10 in]
        n92 = call <vilib>:"Add State(s) to Queue__JKI_lib_State_Machine.vi"("State(s) in (\"\")"=w271) -> ("States Out"=w270:string)  [unwired: 14 in]
      }
      frame "UI: Update When Start" {
        # "Enable: Stop\nDisable: Start, Exit, Settings"
        n93 = Unbundle By Name(w274) -> ("UI Refs.Stop Ref"=w280:refnum<vi>, "UI Refs.Start Ref"=w279:refnum<vi>, "UI Refs.Exit Ref"=w278:refnum<vi>, "UI Refs.Settings Ref"=w277:refnum<vi>, "UI Refs.Data Source Ref"=w273:refnum<vi>)
        n94 = property on="WaveformGraph" class="WFChart (strict)"("History Data"=waveform(dbl)[][] []) -> ()  [unwired: 2 in, 2 out]
        n95 = Build Array(w279, w278, w277, w273) -> (w282:refnum<vi>[])
        n96 = Build Array(w280) -> (w281:refnum<vi>[])
        n97 = call "Set Enable State on Multiple Controls.vi"("Enable?"=TRUE, "Controls"=w281) -> ()  [unwired: 10 in]
        n98 = call "Set Enable State on Multiple Controls.vi"("Enable?"=FALSE, "Controls"=w282) -> ()  [unwired: 10 in]
      }
      frame "UI: Update When Stop" {
        # "Enable: Start, Exit, Settings\nDisable: Stop"
        n99 = Unbundle By Name(w287) -> ("UI Refs.Stop Ref"=w292:refnum<vi>, "UI Refs.Start Ref"=w293:refnum<vi>, "UI Refs.Exit Ref"=w294:refnum<vi>, "UI Refs.Settings Ref"=w295:refnum<vi>, "UI Refs.Data Source Ref"=w286:refnum<vi>)
        n100 = Build Array(w293, w294, w295, w286) -> (w290:refnum<vi>[])
        n101 = Build Array(w292) -> (w291:refnum<vi>[])
        n102 = call "Set Enable State on Multiple Controls.vi"("Enable?"=FALSE, "Controls"=w291) -> ()  [unwired: 10 in]
        n103 = call "Set Enable State on Multiple Controls.vi"("Enable?"=TRUE, "Controls"=w290) -> ()  [unwired: 10 in]
      }
      frame "UI: Cursor Set" {
        # "Argument"
        # "Set and Unset Cursor Busy.\n(Usage: \"UI: Cursor Set >> Busy|Idle\")"
        n104 = disable-structure shown="Default" {
          disable-tunnel: w302 -> [w308 w313]
          disable-tunnel: [w307 w313] -> w301
          disable-tunnel: w300 -> [w306 _]
          frame condition #0 (active) {
            n105 = case shown="\"Busy\"" w306 {
              tunnel: w308 -> [w310 w312]
              tunnel: [w309 w311] -> w307
              frame "Idle", Default {
                n106 = call <vilib>:"Unset Busy.vi"("error in (no error)"=w310) -> ("error out"=w309:errorcluster)  [unwired: 10 in]
              }
              frame "Busy" {
                n107 = call <vilib>:"Set Busy.vi"("error in (no error)"=w312) -> ("error out"=w311:errorcluster)  [unwired: 9 in, 1 out]
              }
            }
          }
          frame condition #1 {
          }
        }
        n108 = call <vilib>:"Add State(s) to Queue__JKI_lib_State_Machine.vi"("State(s) in (\"\")"=w305) -> ("States Out"=w304:string)  [unwired: 14 in]
      }
      frame "UI: Front Panel State" {
        # "Argument"
        # "Set Front Panel Open or Closed\n(Usage: \"UI: Front Panel State >> Open|Close\")"
        n109 = Unbundle By Name(w317) -> ("Core.Current VI Reference"=w316:refnum<vi>)
        n110 = case shown="\"Minimize\", \"Minimized\"" w315 {
          tunnel: w319 -> [w327 w342 w353 w366 w379]
          tunnel: [w329 w343 w355 w368 w381] -> w318
          tunnel: w316 -> [w328 w340 w354 w367 w380]
          frame "Open", "Standard", Default {
            w322 = T2."Standard" ("State")
            n111 = property class="VI"(reference=w328, error in=w327) -> (reference out=w325:refnum<vi>, error out=w326:errorcluster, "FP.State"=w324:T2)
            n112 = Not Equal?(x=w324, y=w322) -> (x != y?=w323:bool)
            n113 = case shown="True" w323 {
              tunnel: [w333 w335] -> w329
              tunnel: w326 -> [w332 w335]
              tunnel: w325 -> [w331 _]
              tunnel: w322 -> [w330 _]
              frame True {
                n114 = invoke class="VI" method="FP.Open"(reference=w331, error in=w332, "Activate"=TRUE, "State"=w330) -> (error out=w333:errorcluster)  [unwired: 1 in, 4 out]
              }
              frame False {
              }
            }
          }
          frame "Close", "Closed" {
            n115 = property class="VI"(reference=w340, error in=w342) -> (reference out=w339:refnum<vi>, error out=w341:errorcluster, "FP.State"=w337:T2)
            n116 = Not Equal?(x=w337, y=T2."Closed" ("Front Panel Window:State")) -> (x != y?=w336:bool)
            n117 = case shown="True" w336 {
              tunnel: [w344 w347] -> w343
              tunnel: w341 -> [w344 w346]
              tunnel: w339 -> [_ w345]
              frame False {
              }
              frame True {
                n118 = invoke class="VI" method="FP.Close"(reference=w345, error in=w346) -> (error out=w347:errorcluster)  [unwired: 1 in, 2 out]
              }
            }
          }
          frame "Hidden", "Hide" {
            w348 = T2."Hidden" ("State")
            n119 = property class="VI"(reference=w354, error in=w353) -> (reference out=w351:refnum<vi>, error out=w352:errorcluster, "FP.State"=w350:T2)
            n120 = Not Equal?(x=w350, y=w348) -> (x != y?=w349:bool)
            n121 = case shown="True" w349 {
              tunnel: [w359 w360] -> w355
              tunnel: w352 -> [w358 w360]
              tunnel: w351 -> [w357 _]
              tunnel: w348 -> [w356 _]
              frame True {
                n122 = invoke class="VI" method="FP.Open"(reference=w357, error in=w358, "State"=w356) -> (error out=w359:errorcluster)  [unwired: 2 in, 4 out]
              }
              frame False {
              }
            }
          }
          frame "Minimize", "Minimized" {
            w361 = T2."Minimized" ("State")
            n123 = property class="VI"(reference=w367, error in=w366) -> (reference out=w364:refnum<vi>, error out=w365:errorcluster, "FP.State"=w363:T2)
            n124 = Not Equal?(x=w363, y=w361) -> (x != y?=w362:bool)
            n125 = case shown="True" w362 {
              tunnel: [w372 w373] -> w368
              tunnel: w365 -> [w371 w373]
              tunnel: w364 -> [w370 _]
              tunnel: w361 -> [w369 _]
              frame True {
                n126 = invoke class="VI" method="FP.Open"(reference=w370, error in=w371, "State"=w369) -> (error out=w372:errorcluster)  [unwired: 2 in, 4 out]
              }
              frame False {
              }
            }
          }
          frame "Maximize", "Maximized" {
            w374 = T2."Maximized" ("State")
            n127 = property class="VI"(reference=w380, error in=w379) -> (reference out=w377:refnum<vi>, error out=w378:errorcluster, "FP.State"=w376:T2)
            n128 = Not Equal?(x=w376, y=w374) -> (x != y?=w375:bool)
            n129 = case shown="True" w375 {
              tunnel: [w385 w386] -> w381
              tunnel: w378 -> [w384 w386]
              tunnel: w377 -> [w383 _]
              tunnel: w374 -> [w382 _]
              frame True {
                n130 = invoke class="VI" method="FP.Open"(reference=w383, error in=w384, "State"=w382) -> (error out=w385:errorcluster)  [unwired: 2 in, 4 out]
              }
              frame False {
              }
            }
          }
        }
        n131 = call <vilib>:"Add State(s) to Queue__JKI_lib_State_Machine.vi"("State(s) in (\"\")"=w321) -> ("States Out"=w320:string)  [unwired: 14 in]
      }
      frame "UI: Change Waveform Graph Legend Num" {
        n132 = call "Convert API String Arguments to Data.vim"("Type"=u32 0 ("Legend:Number of Rows"), "String"=w390) -> ("error"=w388:errorcluster, "Data"=w391:u32)  [unwired: 6 in]
        n133 = Unbundle By Name(w393) -> ("UI Refs.Data Ref"=w392:refnum<vi>)
        n134 = property class="WFChart (strict)"(reference=w392, error in=w388, "LegNumRows"=w391) -> (error out=w387:errorcluster)  [unwired: 1 out]
      }
      frame "UI: Update Waveform Graph" {
        n135 = call "CSM - Convert Argument to MassData.vim"("Type"=waveform(dbl)[] [] ("Data"), "MassData Argument"=w408) -> ("error out"=w406:errorcluster, "Data"=w402:waveform(dbl)[])  [unwired: 6 in]
        "WaveformGraph" <- w402
        n136 = Array Size(array=w402) -> (size(s)=w399:i32)
        n137 = feedback-in #1(w399) -> ()
        n138 = feedback #1(0) -> (w400:i32)
        n139 = Not Equal?(x=w399, y=w400) -> (x != y?=w396:bool)
        n140 = Format Into String(w399) -> (resulting string=w401:string)  [unwired: 3 in, 1 out]
        n141 = call <vilib>:"Build State String with Arguments__JKI_lib_State_Machine.vi"("Arguments (\"\")"=w401, "State"="UI: Change Waveform Graph Legend Num") -> ("State with Arguments"=w397:string)  [unwired: 4 in]
        n142 = call-poly <userlib>:"Add State(s) to Queue By BOOL++.vi"("TRUE(\"\")"=w397, "Condition"=w396, "State Queue(\"\")"=w404) -> ("Remaining States"=w405:string)  [unwired: 8 in]
      }
      frame "---------- Macro ----------" {
        n143 = call <vilib>:"Add State(s) to Queue__JKI_lib_State_Machine.vi"("State(s) in (\"\")"=w415) -> ("States Out"=w414:string)  [unwired: 14 in]
      }
      frame "Macro: Initialize" {
        w416 = "Data: Initialize\nInitialize Core Data\nEvents: Register\nUI: Initialize\nUI: Front Panel State >> Open\nUI: Change Waveform Graph Legend Num >> 1\nDO: Update Status >> Ready...\n\n//Permanent registrations\nAcquired Waveform@Acquisition >> API: Log@Logging -><register>\nAcquired Waveform@Acquisition >> UI: Update Waveform Graph -><register>"  # Data: Initialize Initialize Core Data Events: Register UI: Initialize UI: Front Panel State >> Open UI: Change Waveform Graph Legend Num >> 1 DO: Update Status >> Ready...  //Permanent registrations Acquired Waveform@Acquisition >> API: Log@Logging -><register> Acquired Waveform@Acquisition >> UI: Update Waveform Graph -><register>
        # "Initialization Macro\n(This is called once, when the VI starts)"
        n144 = call <userlib>:"CSM - Populate Configuration Variables.vi"("String in"=w416) -> ("String out"=w417:string)  [unwired: 7 in, 1 out]
        n145 = call <vilib>:"Add State(s) to Queue__JKI_lib_State_Machine.vi"("State(s) in Front (\"\")"=w417, "State(s) in (\"\")"=w422) -> ("States Out"=w421:string)  [unwired: 13 in]
      }
      frame "Macro: Start" {
        n146 = Bundle By Name(cluster=w427, "State"=UI_State."Acquiring and Logging" ("UI State")) -> (w426:T8)
        n147 = call <vilib>:"Add State(s) to Queue__JKI_lib_State_Machine.vi"("State(s) in Front (\"\")"="//Local States\nDO: Update Status >> Acquiring and Logging...\nUI: Update When Start\n\n//Send Message to Other CSM Modules\nAPI: Start -@ Logging\nAPI: Start ->| Acquisition" ("State(s) in Front (\"\")"), "State(s) in (\"\")"=w424) -> ("States Out"=w425:string)  [unwired: 13 in]
      }
      frame "Macro: Stop" {
        n148 = Unbundle By Name(w431) -> ("State"=w433:T4)
        n149 = case shown="Default" w433 {
          selector: w433 -> [w440 _]
          tunnel: [w440 UI_State."Waiting for Stop" ("UI State")] -> w432
          frame "Waiting for Exit" {
          }
          frame Default {
          }
        }
        n150 = Bundle By Name(cluster=w431, "State"=w432) -> (w437:T8)
        n151 = call <vilib>:"Add State(s) to Queue__JKI_lib_State_Machine.vi"("State(s) in Front (\"\")"="//Local States\nDO: Update Status >> Stopping...\nUI: Update When Stop\n\n//Send Message to Other CSM Modules\nAPI: Stop -@ Acquisition\nAPI: Stop -@ Logging\n" ("State(s) in Front (\"\")"), "State(s) in (\"\")"=w435) -> ("States Out"=w436:string)  [unwired: 13 in]
      }
      frame "Macro: Exit" {
        w448 = "UI: Front Panel State >> Close"  # UI: Front Panel State >> Close
        w445 = "//Permanent registrations\nAcquired Waveform@Acquisition >> API: Log@Logging -><unregister>\nAcquired Waveform@Acquisition >> UI: Update Waveform Graph -><unregister>\n\nData: Cleanup\nEvents: Unregister\nExit"  # //Permanent registrations Acquired Waveform@Acquisition >> API: Log@Logging -><unregister> Acquired Waveform@Acquisition >> UI: Update Waveform Graph -><unregister>  Data: Cleanup Events: Unregister Exit
        # "Exit Macro\n(This is called once, when the VI exits)"
        n152 = Unbundle By Name(w450) -> ("Core.Close Panel on Exit?"=w449:bool)
        n153 = disable-structure shown="Disabled" {
          disable-tunnel: [w453 w465] -> w442
          frame Disabled {
            w460 = "Macro: Exit -@ Acquisition\nMacro: Exit -@ Logging"  # Macro: Exit -@ Acquisition Macro: Exit -@ Logging
            n154 = call <userlib>:"CSM - Module Status.vi"("CSM Name"="Algorithm") -> ("#Instance"=w456:i32, "CSM Name(dup)"=w458:string)  [unwired: 6 in, 3 out]
            n155 = for {
              N: w456 -> [_]
              tunnel: w458 -> [w463]
              tunnel: "Macro: Exit" -> [w462]
              tunnel: [w461] -> w454 mode=indexing
              n156 = call-poly <userlib>:"Build Message with Arguments++.vi"("State with Arguments"=w462, "Target Module (\"\")"=w463) -> ("CSM Message String"=w461:string)  [unwired: 13 in]
            }
            n157 = Build Array (concatenate)(w460, w454) -> (w455:string[])
            n158 = call <userlib>:"CSM - Compact Multiple States.vi"("Multiple States"=w455) -> ("States"=w453:string)  [unwired: 9 in]
          }
          frame Enabled {
            # "#NOTE\nHelper VI is equivalent to other case"
            n159 = call <userlib>:"CSM - Build Exit Messages of CSMs.vi"("State with Arguments(\"Macro: Exit“)"="Macro: Exit" ("State with Arguments(\"Macro: Exit“)"), "CSMs"=string[] ["Acquisition", "Logging", "Algorithm"]) -> ("States"=w465:string)  [unwired: 13 in]
          }
        }
        n160 = Select(t=w448, s=w449, f="") -> (s? t:f=w446:string)
        n161 = call <vilib>:"Add State(s) to Queue__JKI_lib_State_Machine.vi"("State(s) in Front (\"\")"=w442, "State(s) in (\"\")"=w446, "State(s) at Back (\"\")"=w445) -> ("States Out"=w444:string)  [unwired: 12 in]
        n162 = call <vilib>:"Add State(s) to Queue__JKI_lib_State_Machine.vi"("State(s) in Front (\"\")"=w444, "State(s) in (\"\")"=w452) -> ("States Out"=w451:string)  [unwired: 13 in]
      }
      frame "---------- DoSth ----------" {
        n163 = call <vilib>:"Add State(s) to Queue__JKI_lib_State_Machine.vi"("State(s) in (\"\")"=w471) -> ("States Out"=w470:string)  [unwired: 14 in]
      }
      frame "Do: Update Status" {
        n164 = call <vilib>:"Add State(s) to Queue__JKI_lib_State_Machine.vi"("State(s) in (\"\")"=w477) -> ("States Out"=w476:string)  [unwired: 14 in]
        "Status" <- w472
      }
      frame "Do: Launch Settings Dialog" {
        # "Your code here.\n(You can make a copy of, or modify, this frame)"
        n165 = call <userlib>:"CSM - Check If Module Exists.vi"("CSM Name"="Acquisition" ("Name(\"\" to use uuid)")) -> ("Error out"=w484:errorcluster, "Exist?"=w480:bool, "CSM Name(dup)"=w482:string)  [unwired: 8 in]
        n166 = case shown="True" w480 {
          tunnel: w484 -> [w492 w504]
          tunnel: w482 -> [w488 w503]
          tunnel: w481 -> [_ w502]
          tunnel: [w491 w501] -> w479
          frame False {
            n167 = Format Into String(format string="Cannot Find the CSM which named %s !!!", w488) -> (resulting string=w487:string)  [unwired: 2 in, 1 out]
            n168 = Bundle By Name(cluster=w492, "status"=TRUE, "source"=w487) -> (w491:errorcluster)
          }
          frame True {
            w496 = T2."Standard" ("State")
            n169 = call <userlib>:"CSM - Module VI Reference.vi"("Current Module(\"\" to generate a ID)"=w502, "error in (no error)"=w504, "force?(F)"=TRUE, "CSM Name"=w503) -> ("error out"=w494:errorcluster, "CSM Module VIRef"=w495:refnum<vi>)  [unwired: 6 in]
            n170 = property class="VI"(reference=w495, error in=w494) -> (reference out=w499:refnum<vi>, error out=w500:errorcluster, "FP.State"=w498:T2)
            n171 = Not Equal?(x=w498, y=w496) -> (x != y?=w497:bool)
            n172 = case shown="True" w497 {
              tunnel: [w511 w513] -> w501
              tunnel: w500 -> [w506 w513]
              tunnel: w499 -> [w505 _]
              tunnel: w496 -> [w510 _]
              frame True {
                n173 = property class="VI"(reference=w505, error in=w506, "FP.Behavior"=T5."Modal" ("Front Panel Window:Behavior")) -> (reference out=w508:refnum<vi>, error out=w509:errorcluster)
                n174 = invoke class="VI" method="FP.Open"(reference=w508, error in=w509, "Activate"=TRUE, "State"=w510) -> (error out=w511:errorcluster)  [unwired: 1 in, 4 out]
              }
              frame False {
              }
            }
          }
        }
      }
      frame "Do: Confirm Quit" {
        n175 = Unbundle By Name(w518) -> ("State"=w521:T4)
        n176 = case shown="Default" w521 {
          tunnel: [UI_State."Idle" ("UI State") w530] -> w520
          tunnel: w518 -> [w525 w529]
          tunnel: [w525 w528] -> w519
          tunnel: [TRUE w527] -> w514
          frame Default {
          }
          frame "Acquiring and Logging" {
            n177 = Two Button Dialog(message="Are you sure you want to quit while the acquisition is running?" ("Confirm Quit Message"), 1:"No" ("No"), 2:"Yes" ("Yes")) -> (T button?=w531:bool)
            n178 = case shown="False" w531 {
              tunnel: [UI_State."Acquiring and Logging" ("UI State") UI_State."Waiting for Exit" ("UI State")] -> w530
              tunnel: w529 -> [w535 w538]
              tunnel: [w535 w538] -> w528
              tunnel: [_ TRUE] -> w527
              frame False {
                # "User did not want to quit."
              }
              frame True {
              }
            }
          }
        }
        n179 = Bundle By Name(cluster=w519, "State"=w520) -> (w517:T8)
        n180 = call-poly <userlib>:"Add State(s) to Queue By BOOL++.vi"("TRUE(\"\")"="Macro: Exit", "Condition"=w514, "State Queue(\"\")"=w523) -> ("Remaining States"=w516:string)  [unwired: 8 in]
      }
    }
  }
  n181 = call <userlib>:"CSM - Sync Configuration Variables to File.vi"("All Temp Variable to Default Ini(F)"=TRUE, "error in (no error)"=w2) -> ("error out"=→"error out":errorcluster)  [unwired: 7 in]
